vi "UHR-Fleezers Control (host) - 11.9b.vi"() -> ()   [LabVIEW 2014] (continued)
                                n672 = Multiply(x=w983, y=w984) -> (x*y=w982:dbl)
                                n673 = Round Toward -Infinity(1:w982) -> (0:w981:dbl)
                                n674 = Select(t=w981, s="Random Choice", f=w987) -> (s? t:f=w985:dbl)
                                n675 = Select(t="Yank to Trap D (MHz)", s="Yank to which?", f="Yank to SP") -> (s? t:f=w978:dbl[])
                                n676 = Index Array(array=w978, index=w985) -> (element=w988:dbl)
                                n677 = case shown="False" "Yank to which?" {
                                tunnel: w988 -> [w989 w1016]
                                frame False {
                                n678 = flat-sequence {
                                tunnel: w989 -> [w990]
                                frame #0 {
                                n679 = property on="Trap Pos FB SP" class="DigNum (strict)"("Val(Sgnl)"=w990) -> ()  [unwired: 2 in, 2 out]
                                }
                                frame #1 {
                                n680 = Wait (ms)(milliseconds to wait=u32 700) -> ()  [unwired: 1 out]
                                }
                                frame #2 {
                                n681 = local read "Action (%)"() -> (w995:dbl)
                                n682 = Absolute Value(x=w995) -> (abs(x)=w994:dbl)
                                n683 = Greater?(x=w994, y=70.0) -> (0:w992:bool)
                                n684 = property on="Remove Action Offset" class="Bool (strict)"("Val(Sgnl)"=w992) -> ()  [unwired: 2 in, 2 out]
                                }
                                frame #3 {
                                n685 = for {
                                N: 4 -> [_]
                                n686 = flat-sequence {
                                frame #0 {
                                n687 = Wait (ms)(milliseconds to wait=u32 500) -> ()  [unwired: 1 out]
                                }
                                frame #1 {
                                n688 = local read "Action (%)"() -> (w1001:dbl)
                                n689 = Absolute Value(x=w1001) -> (abs(x)=w1000:dbl)
                                n690 = Greater?(x=w1000, y=70.0) -> (0:w998:bool)
                                n691 = property on="Remove Action Offset" class="Bool (strict)"("Val(Sgnl)"=w998) -> ()  [unwired: 2 in, 2 out]
                                }
                                }
                                }
                                }
                                frame #4 {
                                n692 = local read "Shift confocal"() -> (w1005:bool)
                                n693 = local read "Mean"() -> (w1008:dbl)
                                n694 = Greater?(x=w1008, y=11.0) -> (0:w1004:bool)
                                n695 = Not(x=w1004) -> (.not. x?=w1003:bool)
                                n696 = And(x=w1003, y=w1005) -> (x .and. y?=w1002:bool)
                                n697 = And(x=w1004, y=w1005) -> (x .and. y?=w1006:bool)
                                n698 = case shown="True" w1006 {
                                frame False {
                                }
                                frame True {
                                n699 = local read "Confocal X 2 (V)"() -> (w1011:dbl)
                                n700 = local read "Confocal Y 2 (V)"() -> (w1012:dbl)
                                n701 = property on="AO2" class="Slide (strict)"("Val(Sgnl)"=w1011) -> ()  [unwired: 2 in, 2 out]
                                n702 = property on="AO1" class="Slide (strict)"("Val(Sgnl)"=w1012) -> ()  [unwired: 2 in, 2 out]
                                }
                                }
                                n703 = case shown="True" w1002 {
                                frame False {
                                }
                                frame True {
                                n704 = local read "Confocal X 1 (V)"() -> (w1009:dbl)
                                n705 = local read "Confocal Y 1 (V)"() -> (w1010:dbl)
                                n706 = property on="AO1" class="Slide (strict)"("Val(Sgnl)"=w1010) -> ()  [unwired: 2 in, 2 out]
                                n707 = property on="AO2" class="Slide (strict)"("Val(Sgnl)"=w1009) -> ()  [unwired: 2 in, 2 out]
                                }
                                }
                                }
                                frame #5 {
                                n708 = Wait (ms)(milliseconds to wait=u32 1500) -> ()  [unwired: 1 out]
                                }
                                frame #6 {
                                n709 = property on="Remove Offset" class="Bool (strict)"("Val(Sgnl)"=TRUE ("Value (Signaling)")) -> ()  [unwired: 2 in, 2 out]
                                n710 = property on="Rem fb disp offset" class="Bool (strict)"("Val(Sgnl)"=TRUE ("Value (Signaling)")) -> ()  [unwired: 2 in, 2 out]
                                }
                                }
                                }
                                frame True {
                                n711 = flat-sequence {
                                tunnel: w1016 -> [w1017]
                                frame #0 {
                                n712 = property on="Trap D (MHz)" class="DigNum (strict)"("Val(Sgnl)"=w1017) -> ()  [unwired: 2 in, 2 out]
                                }
                                frame #1 {
                                n713 = Wait (ms)(milliseconds to wait=u32 500) -> ()  [unwired: 1 out]
                                }
                                frame #2 {
                                n714 = local read "Shift confocal"() -> (w1021:bool)
                                n715 = local read "Mean"() -> (w1019:dbl)
                                n716 = Greater?(x=w1019, y=11.0) -> (0:w1022:bool)
                                n717 = Not(x=w1022) -> (.not. x?=w1023:bool)
                                n718 = And(x=w1023, y=w1021) -> (x .and. y?=w1025:bool)
                                n719 = And(x=w1022, y=w1021) -> (x .and. y?=w1024:bool)
                                n720 = case shown="True" w1024 {
                                frame False {
                                }
                                frame True {
                                n721 = local read "Confocal Y 2 (V)"() -> (w1029:dbl)
                                n722 = local read "Confocal X 2 (V)"() -> (w1028:dbl)
                                n723 = property on="AO1" class="Slide (strict)"("Val(Sgnl)"=w1029) -> ()  [unwired: 2 in, 2 out]
                                n724 = property on="AO2" class="Slide (strict)"("Val(Sgnl)"=w1028) -> ()  [unwired: 2 in, 2 out]
                                }
                                }
                                n725 = case shown="True" w1025 {
                                frame False {
                                }
                                frame True {
                                n726 = local read "Confocal X 1 (V)"() -> (w1026:dbl)
                                n727 = local read "Confocal Y 1 (V)"() -> (w1027:dbl)
                                n728 = property on="AO2" class="Slide (strict)"("Val(Sgnl)"=w1026) -> ()  [unwired: 2 in, 2 out]
                                n729 = property on="AO1" class="Slide (strict)"("Val(Sgnl)"=w1027) -> ()  [unwired: 2 in, 2 out]
                                }
                                }
                                }
                                }
                                }
                                }
                                }
                              }
                            }
                            frame "Raster" {
                              n730 = property on="Trap Raster Scan" class="Bool (strict)"("Val(Sgnl)"=TRUE ("Value (Signaling)")) -> ()  [unwired: 2 in, 2 out]
                            }
                          }
                          n731 = local read "Time (s)"() -> (w962:dbl)
                          "Fl. High" <- TRUE ("Yanking")
                        }
                        frame #1 {
                          n732 = local read "Auto F Reset"() -> (w1031:bool)
                          n733 = case shown="True" w1031 {
                            tunnel: w1036 -> [_ w1040]
                            tunnel: w1035 -> [_ w1039]
                            tunnel: w1034 -> [_ w1038]
                            tunnel: w1032 -> [_ w1037]
                            frame False {
                            }
                            frame True {
                              n734 = node-c288() -> (w1042:T21)  [unwired: 4 out]
                              n735 = timed-loop {
                                timing: w1042 -> [_]
                                timing-out: [_] -> w1041
                                tunnel: w1040 -> [w1060]
                                tunnel: w1039 -> [w1059]
                                tunnel: w1038 -> [w1058]
                                tunnel: w1037 -> [w1057]
                                stop <- w1043 stop-if-true
                                n736 = node-c288() -> ()  [unwired: 2 out]
                                n737 = local read "Fl. D Thresh. (kHz)"() -> (w1051:dbl)
                                n738 = local read "Fl. Triggered..."() -> (w1056:bool)
                                n739 = local read "Delta Fl. 1"() -> (w1047:dbl)
                                n740 = local read "Delta Fl. 2"() -> (w1045:dbl)
                                n741 = local read "Stop All"() -> (w1054:bool)
                                n742 = local read "APD to Watch"() -> (w1046:bool)
                                n743 = Select(t=w1047, s=w1046, f=w1045) -> (s? t:f=w1044:dbl)
                                n744 = Not(x=w1056) -> (.not. x?=w1055:bool)
                                n745 = Multiply(x=w1051, y=1000.0) -> (x*y=w1050:dbl)
                                n746 = Negate(x=w1050) -> (-x=w1049:dbl)
                                n747 = Less?(x=w1044, y=w1049) -> (x < y?=w1053:bool)
                                n748 = Compound Arithmetic op=OR(w1053, w1054, w1055, "Reset Force") -> (w1043:bool)
                                n749 = case shown="True" w1043 {
                                tunnel: w1060 -> [_ w1075]
                                tunnel: w1059 -> [_ w1074]
                                tunnel: w1058 -> [_ w1064]
                                tunnel: w1057 -> [_ w1066]
                                frame False {
                                }
                                frame True {
                                n750 = local read "Time (s)"() -> (w1065:dbl)
                                n751 = case shown="\"Yank\"" w1074 {
                                tunnel: w1075 -> [_ w1078]
                                tunnel: w1066 -> [_ w1076]
                                frame "Image", Default {
                                }
                                frame "Yank" {
                                n752 = flat-sequence {
                                tunnel: [w1084] -> w1079
                                tunnel: w1078 -> [w1084]
                                tunnel: [w1080] -> w1077
                                tunnel: w1076 -> [w1080]
                                tunnel: w1079 -> [w1087]
                                tunnel: w1077 -> [w1085]
                                frame #0 {
                                n753 = local read "Yank Delay (s)"() -> (w1083:dbl)
                                n754 = Multiply(x=w1083, y=1000.0) -> (x*y=w1081:dbl)
                                n755 = Wait (ms)(milliseconds to wait=w1081) -> ()  [unwired: 1 out]
                                }
                                frame #1 {
                                n756 = local read "Yank to which?"() -> (w1086:bool)
                                n757 = case shown="False" w1086 {
                                tunnel: w1087 -> [_ w1115]
                                tunnel: w1085 -> [w1088 _]
                                frame False {
                                n758 = flat-sequence {
                                tunnel: w1088 -> [w1089]
                                frame #0 {
                                n759 = property on="Trap Pos FB SP" class="DigNum (strict)"("Val(Sgnl)"=w1089) -> ()  [unwired: 2 in, 2 out]
                                }
                                frame #1 {
                                n760 = Wait (ms)(milliseconds to wait=u32 700) -> ()  [unwired: 1 out]
                                }
                                frame #2 {
                                n761 = local read "Action (%)"() -> (w1094:dbl)
                                n762 = Absolute Value(x=w1094) -> (abs(x)=w1093:dbl)
                                n763 = Greater?(x=w1093, y=70.0) -> (0:w1091:bool)
                                n764 = property on="Remove Action Offset" class="Bool (strict)"("Val(Sgnl)"=w1091) -> ()  [unwired: 2 in, 2 out]
                                }
                                frame #3 {
                                n765 = for {
                                N: 4 -> [_]
                                n766 = flat-sequence {
                                frame #0 {
                                n767 = Wait (ms)(milliseconds to wait=u32 500) -> ()  [unwired: 1 out]
                                }
                                frame #1 {
                                n768 = local read "Action (%)"() -> (w1100:dbl)
                                n769 = Absolute Value(x=w1100) -> (abs(x)=w1099:dbl)
                                n770 = Greater?(x=w1099, y=70.0) -> (0:w1097:bool)
                                n771 = property on="Remove Action Offset" class="Bool (strict)"("Val(Sgnl)"=w1097) -> ()  [unwired: 2 in, 2 out]
                                }
                                }
                                }
                                }
                                frame #4 {
                                n772 = local read "Shift confocal"() -> (w1105:bool)
                                n773 = local read "Mean"() -> (w1107:dbl)
                                n774 = Greater?(x=w1107, y=11.0) -> (0:w1104:bool)
                                n775 = Not(x=w1104) -> (.not. x?=w1103:bool)
                                n776 = And(x=w1104, y=w1105) -> (x .and. y?=w1102:bool)
                                n777 = And(x=w1103, y=w1105) -> (x .and. y?=w1101:bool)
                                n778 = case shown="True" w1102 {
                                frame False {
                                }
                                frame True {
                                n779 = local read "Confocal Y 2 (V)"() -> (w1111:dbl)
                                n780 = local read "Confocal X 2 (V)"() -> (w1110:dbl)
                                n781 = property on="AO2" class="Slide (strict)"("Val(Sgnl)"=w1110) -> ()  [unwired: 2 in, 2 out]
                                n782 = property on="AO1" class="Slide (strict)"("Val(Sgnl)"=w1111) -> ()  [unwired: 2 in, 2 out]
                                }
                                }
                                n783 = case shown="True" w1101 {
                                frame False {
                                }
                                frame True {
                                n784 = local read "Confocal X 1 (V)"() -> (w1108:dbl)
                                n785 = local read "Confocal Y 1 (V)"() -> (w1109:dbl)
                                n786 = property on="AO1" class="Slide (strict)"("Val(Sgnl)"=w1109) -> ()  [unwired: 2 in, 2 out]
                                n787 = property on="AO2" class="Slide (strict)"("Val(Sgnl)"=w1108) -> ()  [unwired: 2 in, 2 out]
                                }
                                }
                                }
                                frame #5 {
                                n788 = Wait (ms)(milliseconds to wait=u32 1500) -> ()  [unwired: 1 out]
                                }
                                frame #6 {
                                n789 = property on="Rem fb disp offset" class="Bool (strict)"("Val(Sgnl)"=TRUE ("Value (Signaling)")) -> ()  [unwired: 2 in, 2 out]
                                n790 = property on="Remove Offset" class="Bool (strict)"("Val(Sgnl)"=TRUE ("Value (Signaling)")) -> ()  [unwired: 2 in, 2 out]
                                }
                                }
                                }
                                frame True {
                                n791 = flat-sequence {
                                tunnel: w1115 -> [w1116]
                                frame #0 {
                                n792 = property on="Trap D (MHz)" class="DigNum (strict)"("Val(Sgnl)"=w1116) -> ()  [unwired: 2 in, 2 out]
                                }
                                frame #1 {
                                n793 = Wait (ms)(milliseconds to wait=u32 500) -> ()  [unwired: 1 out]
                                }
                                frame #2 {
                                n794 = local read "Shift confocal"() -> (w1122:bool)
                                n795 = local read "Mean"() -> (w1124:dbl)
                                n796 = Greater?(x=w1124, y=11.0) -> (0:w1121:bool)
                                n797 = Not(x=w1121) -> (.not. x?=w1120:bool)
                                n798 = And(x=w1121, y=w1122) -> (x .and. y?=w1119:bool)
                                n799 = And(x=w1120, y=w1122) -> (x .and. y?=w1118:bool)
                                n800 = case shown="True" w1119 {
                                frame False {
                                }
                                frame True {
                                n801 = local read "Confocal Y 2 (V)"() -> (w1128:dbl)
                                n802 = local read "Confocal X 2 (V)"() -> (w1127:dbl)
                                n803 = property on="AO2" class="Slide (strict)"("Val(Sgnl)"=w1127) -> ()  [unwired: 2 in, 2 out]
                                n804 = property on="AO1" class="Slide (strict)"("Val(Sgnl)"=w1128) -> ()  [unwired: 2 in, 2 out]
                                }
                                }
                                n805 = case shown="True" w1118 {
                                frame False {
                                }
                                frame True {
                                n806 = local read "Confocal Y 1 (V)"() -> (w1126:dbl)
                                n807 = local read "Confocal X 1 (V)"() -> (w1125:dbl)
                                n808 = property on="AO2" class="Slide (strict)"("Val(Sgnl)"=w1125) -> ()  [unwired: 2 in, 2 out]
                                n809 = property on="AO1" class="Slide (strict)"("Val(Sgnl)"=w1126) -> ()  [unwired: 2 in, 2 out]
                                }
                                }
                                }
                                }
                                }
                                }
                                }
                                }
                                }
                                }
                                n810 = local read "Messages"() -> (w1073:string)
                                n811 = Subtract(x=w1065, y=w1064) -> (x-y=w1071:dbl)
                                "Duration (s)" <- w1071
                                n812 = Number To Decimal String(number=w1071, width (-)=i16 0) -> (decimal integer string=w1069:string)
                                n813 = Concatenate Strings(w1069, " s fluorescence event." ("string")) -> (w1067:string)
                                n814 = call "Update messages.vi"("Message to add"=w1067, "Old message string"=w1073) -> ("New message string"=w1072:string)
                                n815 = local write "Reset Force"(FALSE ("Reset Force")) -> ()
                                n816 = local write "Waiting"(TRUE ("Waiting")) -> ()
                                n817 = local write "Messages"(w1072) -> ()
                                n818 = local write "Fl. High"(FALSE ("Fl. High")) -> ()
                                n819 = call <vilib>:"Beep.vi"() -> ()  [unwired: 3 in, 9 out]
                                }
                                }
                                n820 = node-c288() -> ()  [unwired: 2 out]
                              }
                              n821 = node-c288(w1041) -> ()  [unwired: 1 out]
                            }
                          }
                        }
                      }
                      n822 = local read "Trap Pos FB SP"() -> (w949:fxp<+/-,16,1>)
                      n823 = local read "Trap D (MHz)"() -> (w954:dbl)
                    }
                  }
                }
                frame #1 {
                  n824 = local read "Stop All"() -> (w1138:bool)
                  n825 = local read "Fl. Triggered..."() -> (w1136:bool)
                  n826 = Not(x=w1136) -> (.not. x?=w1137:bool)
                  n827 = Or(x=w1137, y=w1138) -> (x .or. y?=w1135:bool)
                }
              }
              n828 = case shown="True" w724 {
                frame False {
                }
                frame True {
                  n829 = local read "Confocal Y 1 (V)"() -> (w734:dbl)
                  n830 = local read "Confocal X 1 (V)"() -> (w733:dbl)
                  n831 = property on="AO2" class="Slide (strict)"("Val(Sgnl)"=w733) -> ()  [unwired: 2 in, 2 out]
                  n832 = property on="AO1" class="Slide (strict)"("Val(Sgnl)"=w734) -> ()  [unwired: 2 in, 2 out]
                }
              }
              n833 = case shown="True" w724 {
                frame False {
                }
                frame True {
                  w732 = FALSE ("Fl. High")
                  n834 = local write "Waiting"(w732) -> ()
                  n835 = local write "Fl. High"(w732) -> ()
                }
              }
              n836 = node-c288() -> ()  [unwired: 2 out]
            }
            n837 = node-c288(w722) -> ()  [unwired: 1 out]
          }
        }
      }
      event "Stop All": Value Change {
        n838 = event-data() -> ()  [unwired: 7 out]
        n839 = local read "Stop All"() -> (w1143:bool)
      }
    }
    n840 = node-c288() -> ()  [unwired: 2 out]
  }
  n841 = property on="Saved trap pos" class="WFGraph (strict)"("Visible"=TRUE) -> ()  [unwired: 2 in, 2 out]
  n842 = property on="Trap Delta Graph" class="WFGraph (strict)"("Visible"=FALSE) -> ()  [unwired: 2 in, 2 out]
  n843 = local write "Trap pos"(TRUE ("Trap pos")) -> ()
  n844 = node-c288(2 ("Processor")) -> (w113:T21)  [unwired: 3 out]
  n845 = timed-loop "Control parameters (event loop)" {
    tunnel: w23 -> [w1152]
    shift-right: [w1151] -> _
    shift-left: errorcluster {"status"=FALSE, "code"=0, "source"=""} ("error out") -> [w1150]
    tunnel: [w1149] -> _
    timing: w113 -> [_]
    timing-out: [_] -> w112
    tunnel: w86 -> [w1148]
    tunnel: w27 -> [w1147]
    tunnel: w26 -> [w1146]
    tunnel: w25 -> [w1145]
    tunnel: w24 -> [w1144]
    stop <- w1149 stop-if-true
    n846 = node-c288() -> ()  [unwired: 2 out]
    n847 = event shown="[20] \"Green laser mode\", \"Green ON/Interlacing\": Value Change" {
      selector: _ -> [_ _ _ _ _ _ _ _ _ _ _ _ _ _ _ _ _ _ _ _ _ _ _ _ _ _ _ _ _ _ _ _ _ _ _ _ _ _ _ _ _ _ _ _ _ _ _ _ _ _ _ _ _ _ _ _ _ _ _ _ _ _ _ _ _ _ _ _ _ _ _ _ _ _ _ _ _ _ _ _]
      dyn-events: _ -> [_ _ _ _ _ _ _ _ _ _ _ _ _ _ _ _ _ _ _ _ _ _ _ _ _ _ _ _ _ _ _ _ _ _ _ _ _ _ _ _ _ _ _ _ _ _ _ _ _ _ _ _ _ _ _ _ _ _ _ _ _ _ _ _ _ _ _ _ _ _ _ _ _ _ _ _ _ _ _ _]
      timeout: _ -> [_ _ _ _ _ _ _ _ _ _ _ _ _ _ _ _ _ _ _ _ _ _ _ _ _ _ _ _ _ _ _ _ _ _ _ _ _ _ _ _ _ _ _ _ _ _ _ _ _ _ _ _ _ _ _ _ _ _ _ _ _ _ _ _ _ _ _ _ _ _ _ _ _ _ _ _ _ _ _ _]
      tunnel: w1152 -> [w1190 _ _ _ w1228 _ w1250 _ _ _ _ w1316 _ _ w1359 w1365 w1370 w1376 w1412 w1430 w1439 _ w1456 w1460 w1471 w1482 w1493 w1504 w1515 w1526 w1553 w1647 w1654 w1692 _ _ w1752 w1756 w1767 w1771 w1775 _ w1783 _ _ _ _ _ _ _ _ _ _ _ _ _ _ _ _ _ w2164 _ w2181 _ w2188 w2206 _ w2213 w2221 w2236 w2247 w2253 _ w2262 _ w2281 _ _ _ w2356]
      tunnel: [w1189 _ _ _ w1218 _ w1249 _ _ w1281 _ w1295 _ _ w1358 w1361 w1367 w1373 w1411 w1428 w1438 _ w1454 _ w1465 w1476 w1487 w1498 w1509 w1520 w1551 w1645 w1652 w1690 _ _ w1750 w1754 w1757 w1769 w1773 _ w1781 _ _ _ _ _ _ _ _ _ _ _ _ _ _ _ _ _ w2162 _ _ _ _ w2203 _ _ _ _ _ _ _ _ _ _ _ _ _ w2354] -> w1151
      tunnel: w1150 -> [w1188 _ _ _ w1227 _ w1248 _ _ w1281 _ w1315 _ _ w1357 w1360 w1366 w1372 w1410 w1429 w1437 _ w1455 w1459 w1470 w1481 w1492 w1503 w1514 w1525 w1552 w1646 w1653 w1691 _ _ w1751 w1755 w1766 w1770 w1774 _ w1782 _ _ _ _ _ _ _ _ _ _ _ _ _ _ _ _ _ w2163 _ w2180 _ w2187 w2205 _ w2212 w2220 w2235 w2246 w2252 _ w2261 _ w2280 _ _ _ w2355]
      tunnel: [_ _ _ _ _ _ _ _ _ w1280 _ _ _ _ _ _ _ _ _ _ _ _ _ _ _ _ _ _ _ _ _ _ _ _ _ _ _ _ _ _ _ _ _ _ _ _ _ _ _ _ _ _ _ _ _ _ _ _ _ _ _ _ _ _ _ _ _ _ _ _ _ _ _ _ _ _ _ _ _ _] -> w1149
      tunnel: [_ _ _ _ _ _ _ "Round T1 X" _ _ _ _ _ _ _ _ _ _ _ _ _ _ _ _ _ _ _ _ _ _ _ _ _ _ _ _ _ _ _ _ _ _ _ _ _ _ _ _ _ _ _ _ _ _ _ _ _ _ _ _ _ _ _ _ _ _ _ _ _ _ _ _ _ _ _ _ _ _ _ _] -> _
      tunnel: [_ _ _ "Adjust Scale\nto Mean" _ _ _ _ _ _ _ _ _ _ _ _ _ _ _ _ _ _ "Test ttrig" _ _ _ _ _ _ _ _ _ _ _ _ _ _ _ _ _ _ _ _ _ _ _ _ _ _ _ "Flush Sample" "Flush Pump 3" "Flush Pump 1" "Clear Volume" _ _ _ _ _ _ _ _ _ _ _ _ _ _ _ _ _ _ _ _ _ _ _ _ _ _] -> _
      tunnel: [_ _ _ _ _ _ _ _ "Round T2 X" _ "Delayed Interlace Start" _ _ _ _ _ _ _ _ _ _ _ _ _ _ _ _ _ _ _ _ _ _ _ _ _ _ _ _ _ _ _ _ _ _ _ _ _ _ _ _ _ _ _ _ _ _ _ _ _ _ _ _ _ _ _ _ _ _ _ _ _ _ _ _ _ _ _ _ _] -> _
      tunnel: w1148 -> [_ _ _ _ _ _ _ _ _ _ _ _ _ _ _ _ _ _ _ _ _ _ _ _ _ _ _ _ _ _ _ _ _ _ _ _ _ _ _ _ _ _ _ _ _ _ w1941 w1959 w1966 w1971 w1977 _ _ w2076 _ _ _ _ _ _ _ _ _ _ _ _ _ _ _ _ _ _ _ _ _ _ _ _ _ _]
      tunnel: w1147 -> [_ _ _ _ _ _ _ _ _ _ _ _ _ _ _ _ _ _ _ _ _ _ _ _ _ _ _ _ _ _ _ _ _ _ _ _ _ _ _ _ _ _ _ _ w1857 _ _ _ _ _ _ w2007 _ _ w2083 _ w2092 _ w2106 _ _ _ _ _ _ _ _ _ _ _ _ _ _ _ _ _ _ _ _ _]
      tunnel: w1146 -> [_ _ _ _ _ _ _ _ _ _ _ _ _ _ _ _ _ _ _ _ _ _ _ _ _ _ _ _ _ _ _ _ _ _ _ _ _ _ _ _ _ _ _ _ _ _ _ _ _ _ _ _ _ _ _ _ _ _ _ _ _ _ _ _ _ _ _ _ _ _ _ _ _ _ _ _ _ _ _ _]
      tunnel: w1145 -> [_ _ _ _ _ _ _ _ _ _ _ _ _ _ _ _ _ _ _ _ _ _ _ _ _ _ _ _ _ _ _ _ _ _ _ _ _ _ _ _ _ _ _ w1794 _ _ _ _ _ _ _ _ w2037 _ _ w2088 _ w2099 _ w2131 _ _ _ _ _ _ _ _ _ _ _ _ _ _ _ _ _ _ _ _]
      tunnel: w1144 -> [_ _ _ _ _ _ _ _ _ _ _ _ _ _ _ _ _ _ _ _ _ _ _ _ _ _ _ _ _ _ _ _ _ _ _ _ _ _ _ _ _ _ _ _ _ _ _ _ _ _ _ _ _ _ _ _ _ _ _ _ _ _ _ _ _ _ _ _ _ _ _ _ _ _ _ _ _ _ _ _]
      event "AI Count (ticks)", "Sets to FIFO (Traps)", "Save ave N", "FPGA Ave.", "# Samples/channel", "N sets to save": Value Change {
        # "So that if 'Save ave N' is updated, the AOD scanning code updates too."
        n848 = event-data() -> ()  [unwired: 6 out]
        n849 = local read "AI Count (ticks)"() -> (w1170:u32)
        n850 = Boolean To (0,1)(Boolean="Sets to FIFO (Traps)") -> (0, 1=w1180:cluster{"Set 1":i16, "Set 2":i16, "Set 3":i16})
        n851 = Cluster To Array(cluster=w1180) -> (array=w1179:i16[])
        n852 = xnode "Read/Write Control"("FPGA VI Reference In"=w1190, "error in"=w1188, "ai count"=w1170, "AI1 Sets to FIFO"="Sets to FIFO (Traps)", "N of AI1 Int Acq Sets"="N Acq Sets (Traps + Fl.)") -> ("error out"=w1189:errorcluster)  [unwired: 1 out]
        n853 = To Unsigned Long Integer(number=w1179) -> (unsigned 32bit integer=w1159:u32[])
        n854 = local read "Scan steps (AOD)"() -> (w1181:u64)
        n855 = Multiply(x=w1170, y="N Acq Sets (Traps + Fl.)") -> (x*y=w1168:u32)
        n856 = Divide(x=40000000.0, y=w1170) -> (x/y=w1162:dbl)
        "AI rate (Hz)" <- w1162
        "Ave. Rate (Hz)" <- w1162
        n857 = Add Array Elements(numeric array=w1159) -> (sum=w1171:u32)
        "Trap Sets" <- w1171
        n858 = Reciprocal(x=w1162) -> (1/x=→"Ave. Period (s)":dbl)
        n859 = property on="Scan steps (AOD)" class="DigNum (strict)"("Val(Sgnl)"=w1181) -> ()  [unwired: 2 in, 2 out]
        n860 = Divide(x=w1162, y="N Acq Sets (Traps + Fl.)") -> (x/y=w1185:dbl)
        "Data Rate (Hz)" <- w1185
        n861 = Reciprocal(x=w1185) -> (1/x=→"Data Period (s)":dbl)
        n862 = local read "Save ave N"() -> (w1184:dbl)
        n863 = Divide(x=w1185, y=w1184) -> (x/y=w1183:dbl)
        "Save Data Rate (Hz)" <- w1183
        n864 = Reciprocal(x=w1183) -> (1/x=→"Save Data Period (s)":dbl)
        n865 = Multiply(x=w1168, y="# Samples/trap") -> (x*y=w1166:u32)
        "Counts/DMA" <- w1166
        n866 = property on="Trap Disp. Downsample" class="DigNum (strict)"("Maximum"="# Samples/trap") -> ()  [unwired: 2 in, 2 out]
        n867 = Multiply(x=w1171, y="# Samples/trap") -> (x*y=w1160:u32)
        "# Samples/channel" <- w1160
        n868 = Multiply(x=w1160, y=u32 8) -> (x*y=→"Trap AI Elements/DMA read":u32)
        n869 = local read "APD Int. Count"() -> (w1167:u32)
        n870 = Multiply(x=w1160, y=u32 3) -> (x*y=→"Trap Pos Elements/DMA read":u32)
        n871 = Divide(x=w1166, y=w1167) -> (x/y=w1157:dbl)
        "APD Samples/FIFO Acq." <- w1157
        n872 = Divide(x=w1166, y=40000000.0) -> (x/y=w1164:dbl)
        "DMA Update Period (s)" <- w1164
        n873 = Multiply(x=2.0, y=w1157) -> (x*y=→"APD Elements/DMA read":dbl)
        n874 = property on="APD Disp. Downsample" class="DigNum (strict)"("Maximum"=w1157) -> ()  [unwired: 2 in, 2 out]
        n875 = local read "N sets to save"() -> (w1177:u32)
        n876 = Multiply(x=w1164, y=w1177) -> (x*y=→"Total Time (s)":dbl)
        "FPGA Averaging" <- FALSE ("FPGA Averaging")
      }
      event "Remove Offset": Value Change {
        n877 = event-data() -> ()  [unwired: 7 out]
        n878 = local write "Remove Offset"(FALSE ("Remove Offset")) -> ()
        n879 = local read "Bead Mean (nm)"() -> (w1192:dbl)
        n880 = local read "Offset (nm)"() -> (w1193:dbl)
        n881 = Add(x=w1192, y=w1193) -> (x+y=w1191:dbl)
        n882 = local write "Offset (nm)"(w1191) -> ()
        n883 = disable-structure shown="Disabled" {
          frame Disabled {
            n884 = local read "Bead Mean (nm)"() -> (w1198:dbl)
            n885 = Add(y=w1198) -> (x=w1197:dbl, x+y=w1196:dbl)
            n886 = Subtract(x=w1198, y=w1197) -> (x-y=w1195:dbl)
            n887 = property on="Bead Separation" class="WFChart (strict)"("YScale.Minimum"=w1195) -> ()  [unwired: 2 in, 2 out]
            n888 = property on="Bead Separation" class="WFChart (strict)"("YScale.Maximum"=w1196) -> ()  [unwired: 2 in, 2 out]
          }
          frame Enabled {
          }
        }
      }
      event "Detector Type": Value Change {
        n889 = event-data() -> ()  [unwired: 7 out]
        n890 = local read "AI labels"() -> (w1199:string[])
        n891 = property on="High Res. Display" class="Ring (strict)"("Strings []"=w1199) -> ()  [unwired: 2 in, 2 out]
        n892 = Build Array (concatenate)(w1199, "none") -> (w1200:string[])
        n893 = property on="FFT 1 Choice 1" class="Ring (strict)"("Strings []"=w1200) -> ()  [unwired: 2 in, 2 out]
        n894 = property on="FFT 1 Choice 2" class="Ring (strict)"("Strings []"=w1200) -> ()  [unwired: 2 in, 2 out]
        n895 = property on="FFT 2 Choice 1" class="Ring (strict)"("Strings []"=w1200) -> ()  [unwired: 2 in, 2 out]
        n896 = property on="FFT 2 Choice 2" class="Ring (strict)"("Strings []"=w1200) -> ()  [unwired: 2 in, 2 out]
        n897 = Bundle("APD 1", "APD 2") -> (w1203:cluster{string, string})  [unwired: 1 out]
        n898 = Cluster To Array(cluster=w1203) -> (array=w1201:string[])
        n899 = Build Array (concatenate)(w1201, w1200) -> (w1205:string[])
        n900 = Array Size(array=w1205) -> (size(s)=w1206:i32)
        n901 = property on="Signals to Plot" class="LstBox (strict)"("Item Names"=w1205) -> ()  [unwired: 2 in, 2 out]
        n902 = property on="Signals to Plot" class="LstBox (strict)"("Number of Rows"=w1206) -> ()  [unwired: 2 in, 2 out]
        n903 = property on="All Signals" class="WFChart (strict)"("LegNumRows"=w1206) -> ()  [unwired: 2 in, 2 out]
      }
      event "Adjust Scale\nto Mean": Value Change {
        n904 = event-data() -> ()  [unwired: 7 out]
        n905 = local read "APD 1 Rate (Hz)"() -> (w1215:dbl)
        n906 = Multiply(x=1000.0, y="Above (kHz)") -> (x*y=w1213:dbl)
        n907 = Multiply(x=1000.0, y="Below (kHz)") -> (x*y=w1211:dbl)
        n908 = Add(x=w1213, y=w1215) -> (x+y=w1208:dbl)
        n909 = Subtract(x=w1215, y=w1211) -> (x-y=w1209:dbl)
        n910 = property on="APD Chart" class="WFChart (strict)"("YScale.Minimum"=w1209) -> ()  [unwired: 2 in, 2 out]
        n911 = property on="APD Chart" class="WFChart (strict)"("YScale.Maximum"=w1208) -> ()  [unwired: 2 in, 2 out]
      }
      event "Phase adj. (AI1)", "+ phase (AI1)", "- phase (AI1)": Value Change {
        n912 = event-data() -> ()  [unwired: 7 out]
        n913 = Negate(x="Phase adj. (AI1)") -> (-x=w1225:i16)
        n914 = Select(t=w1225, s="- phase (AI1)", f="Phase adj. (AI1)") -> (s? t:f=w1224:i16)
        n915 = xnode "Read/Write Control"("FPGA VI Reference In"=w1228, "error in"=w1227, "Phase count adjustment"=w1224) -> ("FPGA VI Reference Out"=w1223:T19, "error out"=w1222:errorcluster)
        n916 = Or(x="- phase (AI1)", y="+ phase (AI1)") -> (x .or. y?=w1219:bool)
        n917 = xnode "Read/Write Control"("FPGA VI Reference In"=w1223, "error in"=w1222, "+ phase"=w1219) -> ("error out"=w1218:errorcluster)  [unwired: 1 out]
      }
      event "Signals to Plot": Double Click {
        w1231 = u32 9868950 ("Color Box")
        n918 = event-data() -> ("Row"=w1233:i32)  [unwired: 9 out]
        n919 = property on="All Signals" class="WFChart (strict)"("Active Plot"=w1233) -> (error out=w1244:errorcluster)  [unwired: 2 in, 1 out]
        n920 = property on="All Signals" class="WFChart (strict)" props=["Plot", "Visible?", "Plot", "Plot Color"](error in=w1244) -> (error out=w1243:errorcluster, "Plot.Visible?"=w1242:bool)  [unwired: 1 in, 2 out]
        n921 = Select(t=FALSE ("Plot.Visible"), s=w1242, f=TRUE ("Plot.Visible")) -> (s? t:f=w1237:bool)
        n922 = property on="All Signals" class="WFChart (strict)"(error in=w1243, "Plot.Visible?"=w1237) -> (error out=w1239:errorcluster)  [unwired: 1 in, 1 out]
        n923 = property on="All Signals" class="WFChart (strict)"(error in=w1239) -> (error out=w1234:errorcluster, "Plot.Plot Color"=w1238:u32)  [unwired: 1 in, 1 out]
        n924 = property on="Signals to Plot" class="LstBox (strict)"(error in=w1234, "Active Row"=w1233) -> (error out=w1232:errorcluster)  [unwired: 1 in, 1 out]
        n925 = Select(t=w1238, s=w1237, f=u32 0) -> (s? t:f=w1235:u32)
        n926 = property on="Signals to Plot" class="LstBox (strict)"(error in=w1232, "CellFontColor"=w1235, "SelColor"=w1231, "CellBG"=w1231, "CellFontSize"=u32 20 ("Active Row:Cell Font:Size"), "CellFontBold"=TRUE ("Active Row:Cell Font:Bold")) -> ()  [unwired: 1 in, 2 out]
      }
      event "BD 1 Frequency 1 (MHz)", "BD 1 Frequency 2 (MHz)", "BD 1 Frequency 3 (MHz)", "BD 2 Frequency 1 (MHz)", "BD 2 Frequency 2 (MHz)", "BD 2 Frequency 3 (MHz)", "Trap D (MHz)": Value Change {
        n927 = event-data() -> ("CtlRef"=w1247:refnum<vi>)  [unwired: 6 out]
        n928 = control-ref of="Trap D (MHz)"() -> (w1246:refnum<vi>)
        n929 = Equal?(x=w1246, y=w1247) -> (x = y?=w1245:bool)
        n930 = case shown="False" "Oscillate Set 1" {
          tunnel: w1250 -> [w1270 _]
          tunnel: [w1269 w1273] -> w1249
          tunnel: w1248 -> [w1268 w1273]
          tunnel: w1245 -> [w1253 _]
          frame False {
            n931 = local read "BD 1 Frequency 2 (MHz)"() -> (w1257:dbl)
            n932 = local read "BD 1 Frequency 1 (MHz)"() -> (w1255:dbl)
            n933 = Subtract(x=w1257, y="Trap D (MHz)") -> (x-y=w1254:dbl)
            n934 = Select(t=w1254, s=w1253, f=w1255) -> (s? t:f=w1252:dbl)
            n935 = local read "Y RF Frequency Limits (MHz)"() -> (w1258:T16)
            n936 = local read "X RF Frequency Limits (MHz)"() -> (w1259:T16)
            n937 = local read "BD 1 Frequency 3 (MHz)"() -> (w1271:dbl)
            n938 = local write "BD 1 Frequency 1 (MHz)"(w1252) -> ()
            n939 = local read "BD 2 Frequency 1 (MHz)"() -> (w1262:dbl)
            n940 = local read "BD 2 Frequency 2 (MHz)"() -> (w1261:dbl)
            n941 = local read "BD 2 Frequency 3 (MHz)"() -> (w1272:dbl)
            n942 = call "set RF board frequency - interlace.vi"("Board 2 Frequency Limits"=w1258, "Board 1 Frequency Limits"=w1259, "error in"=w1268, "FPGA VI Reference In"=w1270, "Board 2 Frequency 3 (MHz)"=w1272, "Board 1 Frequency 3 (MHz)"=w1271, "Board 2 Frequency 2 (MHz)"=w1261, "Board 2 Frequency 1 (MHz)"=w1262, "Board 1 Frequency 2 (MHz)"=w1257, "Board 1 Frequency 1  (MHz)"=w1252) -> ("error out"=w1269:errorcluster)  [unwired: 1 out]
            n943 = Subtract(x=w1262, y=w1261) -> (x-y=w1266:dbl)
            n944 = Subtract(x=w1252, y=w1257) -> (x-y=w1267:dbl)
            n945 = Square(x=w1266) -> (x^2=w1264:dbl)
            n946 = Square(x=w1267) -> (x^2=w1265:dbl)
            n947 = Add(x=w1265, y=w1264) -> (x+y=w1263:dbl)
            n948 = Square Root(x=w1263) -> (sqrt(x)=w1260:dbl)
            n949 = local write "Trap D (MHz)"(w1260) -> ()
            n950 = property on="Initial D (MHz)" class="DigNum (strict)"("Val(Sgnl)"=w1260) -> ()  [unwired: 2 in, 2 out]
          }
          frame True {
          }
        }
      }
      event "Round T1 X": Value Change {
        n951 = event-data() -> ()  [unwired: 7 out]
        n952 = local read "BD 1 Frequency 1 (MHz)"() -> (w1276:dbl)
        n953 = Round To Nearest(number=w1276) -> (nearest integer value=w1275:dbl)
        n954 = property on="BD 1 Frequency 1 (MHz)" class="DigNum (strict)"("Val(Sgnl)"=w1275) -> ()  [unwired: 2 in, 2 out]
      }
      event "Round T2 X": Value Change {
        n955 = event-data() -> ()  [unwired: 7 out]
        n956 = local read "BD 1 Frequency 2 (MHz)"() -> (w1278:dbl)
        n957 = Round To Nearest(number=w1278) -> (nearest integer value=w1277:dbl)
        n958 = property on="BD 1 Frequency 2 (MHz)" class="DigNum (strict)"("Val(Sgnl)"=w1277) -> ()  [unwired: 2 in, 2 out]
      }
      event "Stop All": Value Change {
        n959 = event-data() -> ()  [unwired: 7 out]
        n960 = local read "Stop All"() -> (w1280:bool)
      }
      event "Delayed Interlace Start": Value Change {
        n961 = event-data() -> ()  [unwired: 7 out]
        n962 = flat-sequence {
          frame #0 {
            n963 = Multiply(x="Delay to Interlace (s)", y=1000.0) -> (x*y=w1283:dbl)
            n964 = Wait (ms)(milliseconds to wait=w1283) -> ()  [unwired: 1 out]
          }
          frame #1 {
            n965 = property on="Green laser mode" class="RadioBtnsControl (strict)"("Val(Sgnl)"=enum32{"Laser ON", "Laser OFF", "Interlace"}."Interlace" ("Value (Signaling)")) -> ()  [unwired: 2 in, 2 out]
          }
        }
      }
      event "BD 1 Amplitude 1 (%)", "BD 1 Amplitude 2 (%)", "BD 1 Amplitude 3 (%)", "BD 2 Amplitude 1 (%)", "BD 2 Amplitude 2 (%)", "BD 2 Amplitude 3 (%)", "Trap 1 ON", "Trap 2 ON", "Trap 3 ON", "Feedback On/Off", "All FB On/Off": Value Change {
        w1307 = i16 1 ("f")
        n966 = event-data() -> ()  [unwired: 7 out]
        n967 = local write "Trap 1 (ON/OFF)"("Trap 1 ON") -> ()
        n968 = local write "Trap 2 (ON/OFF)"("Trap 2 ON") -> ()
        n969 = Boolean To (0,1)(Boolean="Trap 3 ON") -> (0, 1=w1308:i16)
        n970 = Boolean To (0,1)(Boolean="Trap 1 ON") -> (0, 1=w1309:i16)
        n971 = Boolean To (0,1)(Boolean="Trap 2 ON") -> (0, 1=w1310:i16)
        n972 = Select(t=w1310, s="Trap ON/OFF X or Y Amp?", f=w1307) -> (s? t:f=w1305:i16)
        n973 = Select(t=w1309, s="Trap ON/OFF X or Y Amp?", f=w1307) -> (s? t:f=w1306:i16)
        n974 = Select(t=w1308, s="Trap ON/OFF X or Y Amp?", f=w1307) -> (s? t:f=w1304:i16)
        n975 = Select(t=w1307, s="Trap ON/OFF X or Y Amp?", f=w1310) -> (s? t:f=w1302:i16)
        n976 = Select(t=w1307, s="Trap ON/OFF X or Y Amp?", f=w1309) -> (s? t:f=w1303:i16)
        n977 = Select(t=w1307, s="Trap ON/OFF X or Y Amp?", f=w1308) -> (s? t:f=w1301:i16)
        n978 = And(x="All FB On/Off", y="Feedback On/Off") -> (x .and. y?=w1299:cluster{"Set 1":bool, "Set 2":bool})
        n979 = local read "BD 1 Amplitude 1 (%)"() -> (w1319:dbl)
        n980 = local read "BD 1 Amplitude 2 (%)"() -> (w1318:dbl)
        n981 = local read "BD 1 Amplitude 3 (%)"() -> (w1317:dbl)
        n982 = Unbundle By Name(w1299) -> ("Set 1"=w1294:bool, "Set 2"=w1291:bool)
        n983 = local read "Y RF Amplitude Limits (%)"() -> (w1287:T16)
        n984 = local read "X RF Amplitude Limits (%)"() -> (w1288:T16)
        n985 = local read "BD 2 Amplitude 1 (%)"() -> (w1320:dbl)
        n986 = local read "BD 2 Amplitude 2 (%)"() -> (w1321:dbl)
        n987 = local read "BD 2 Amplitude 3 (%)"() -> (w1322:dbl)
        n988 = And(x="Trap 2 ON", y=w1291) -> (x .and. y?=w1289:bool)
        n989 = And(x="Trap 1 ON", y=w1294) -> (x .and. y?=w1292:bool)
        n990 = Multiply(x=w1306, y=w1319) -> (x*y=w1314:dbl)
        n991 = Multiply(x=w1318, y=w1305) -> (x*y=w1312:dbl)
        n992 = Multiply(x=w1317, y=w1304) -> (x*y=w1313:dbl)
        n993 = Multiply(x=w1320, y=w1303) -> (x*y=w1323:dbl)
        n994 = Multiply(x=w1321, y=w1302) -> (x*y=w1324:dbl)
        n995 = Multiply(x=w1322, y=w1301) -> (x*y=w1325:dbl)
        n996 = call "set RF board amplitude - interlace.vi"("Board 2 Amplitude Limits"=w1287, "Board 1 Amplitude Limits"=w1288, "error in"=w1315, "FPGA VI Reference In"=w1316, "Board 2 Amplitude 3 (%)"=w1325, "Board 1 Amplitude 3 (%)"=w1313, "Board 2 Amplitude 2 (%)"=w1324, "Board 2 Amplitude 1 (%)"=w1323, "Board 1 Amplitude 2 (%)"=w1312, "Board 1 Amplitude 1 (%)"=w1314) -> ("error out"=w1296:errorcluster, "FPGA VI Reference Out"=w1297:T19)
        n997 = xnode "Read/Write Control"("FPGA VI Reference In"=w1297, "error in"=w1296, "FB On/Off Set 1"=w1292, "FB On/Off Set 2"=w1289) -> ("error out"=w1295:errorcluster)  [unwired: 1 out]
      }
      event "Load parameters": Value Change {
        n998 = event-data() -> ()  [unwired: 7 out]
        n999 = property on="Saved AOD Raster Scan Parameter Sets" class="Arr (strict)"() -> ("Index Values"=w1336:u32[])  [unwired: 2 in, 2 out]
        n1000 = Index Array(array=w1336, index=0) -> (element=w1333:u32)
        n1001 = local write "Load parameters"(FALSE ("Load parameters")) -> ()
        n1002 = Index Array(array="Saved AOD Raster Scan Parameter Sets", index=w1333) -> (element=w1332:T26)
        n1003 = Unbundle By Name(w1332) -> ("Scan Range AOD (nm) 2"=w1331:dbl, "Step Size AOD (nm) 2"=w1330:dbl, "Scan Speed AOD (nm/s) 2"=w1329:dbl, "Number of scans (AOD) 2"=w1328:u16)
        n1004 = flat-sequence {
          tunnel: w1331 -> [w1339]
          tunnel: w1330 -> [w1338]
          tunnel: w1329 -> [w1337]
          tunnel: w1328 -> [w1340]
          frame #0 {
            n1005 = local write "Scan Speed (nm/s)"(w1337) -> ()
            n1006 = local write "Scan Range (nm)"(w1339) -> ()
            n1007 = local write "Step Size (nm)"(w1338) -> ()
          }
          frame #1 {
            n1008 = property on="Number of F/B Scans (AOD)" class="DigNum (strict)"("Val(Sgnl)"=w1340) -> ()  [unwired: 2 in, 2 out]
          }
        }
      }
      event "Trap 1 (ON/OFF)", "Trap 2 (ON/OFF)": Value Change {
        n1009 = event-data() -> ()  [unwired: 7 out]
        n1010 = property on="Trap 2 ON" class="Bool (strict)"("Val(Sgnl)"="Trap 2 (ON/OFF)") -> ()  [unwired: 2 in, 2 out]
        n1011 = property on="Trap 1 ON" class="Bool (strict)"("Val(Sgnl)"="Trap 1 (ON/OFF)") -> ()  [unwired: 2 in, 2 out]
      }
      event "DIO count 1 (ticks)", "DIO count 2 (ticks)", "DIO count 3 (ticks)", "Interlace", "Number Interlace Sets", "Not-Interlacing Set": Value Change {
        n1012 = event-data() -> ()  [unwired: 7 out]
        n1013 = local read "DIO count 3 (ticks)"() -> (w1353:u32)
        n1014 = local read "DIO count 1 (ticks)"() -> (w1355:u32)
        n1015 = local read "DIO count 2 (ticks)"() -> (w1354:u32)
        n1016 = To Unsigned Byte Integer(number="Not-Interlacing Set") -> (unsigned 8bit integer=w1344:u8)
        n1017 = Add(x=w1344, y=u8 1) -> (x+y=w1348:u8)
        n1018 = xnode "Read/Write Control"("FPGA VI Reference In"=w1359, "error in"=w1357, "DIO count 1 (ticks)"=w1355, "DIO count 2 (ticks)"=w1354, "DIO count 3 (ticks)"=w1353, "Interlace ON/OFF"="Interlace", "Number Interlace Cycles"="Number Interlace Sets", "Interlace Off Parameters"=w1348) -> ("error out"=w1358:errorcluster)  [unwired: 1 out]
        n1019 = Build Array(w1355, w1354, w1353) -> (w1346:u32[])
        n1020 = Split 1D Array(array=w1346, index="Number Interlace Sets") -> (first subarray=w1356:u32[])  [unwired: 1 out]
        n1021 = Index Array(array=w1346, index=w1344) -> (element=w1345:u32)
        n1022 = Add Array Elements(numeric array=w1356) -> (sum=w1350:u32)
        n1023 = Select(t=w1350, s="Interlace", f=w1345) -> (s? t:f=→"Total Counts (ticks)":u32)
      }
      event "Reset Feedback": Value Change {
        n1024 = event-data() -> ()  [unwired: 7 out]
        n1025 = Unbundle By Name("Reset Feedback") -> ("Set 1"=w1363:bool, "Set 2"=w1362:bool)
        n1026 = xnode "Read/Write Control"("FPGA VI Reference In"=w1365, "error in"=w1360, "FB Reset Set 1"=w1363, "FB Reset Set 2"=w1362) -> ("error out"=w1361:errorcluster)  [unwired: 1 out]
      }
      event "PID Gains": Value Change {
        n1027 = event-data() -> ()  [unwired: 7 out]
        n1028 = Unbundle By Name("PID Gains") -> ("Set 1"=w1369:T14, "Set 2"=w1368:T14)
        n1029 = xnode "Read/Write Control"("FPGA VI Reference In"=w1370, "error in"=w1366, "FB Gains Set 1"=w1369, "FB Gains Set 2"=w1368) -> ("error out"=w1367:errorcluster)  [unwired: 1 out]
      }
      event "AI2 to Setpoint", "Setpoints (V)": Value Change {
        n1030 = event-data() -> ()  [unwired: 7 out]
        n1031 = xnode "Read/Write Control"("FPGA VI Reference In"=w1376, "error in"=w1372) -> ("FPGA VI Reference Out"=w1375:T19, "error out"=w1374:errorcluster, "AI2 Y Sum Set 1"=w1383:i16, "AI2 Y Sum Set 2"=w1382:i16)
        n1032 = Cluster To Array(cluster="AI2 to Setpoint") -> (array=w1386:bool[])
        n1033 = local read "AI2 (V)"() -> (w1384:cluster{"Set 1":dbl, "Set 2":dbl})
        n1034 = Or Array Elements(Boolean array=w1386) -> (logical OR=w1387:bool)
        n1035 = Bundle By Name(cluster=w1384, "Set 1"=w1383, "Set 2"=w1382) -> (w1381:cluster{"Set 1":dbl, "Set 2":dbl})
        n1036 = Divide(x=w1381, y=3276.7) -> (x/y=w1380:cluster{"Set 1":dbl, "Set 2":dbl})
        "AI2 (V)" <- w1380
        n1037 = case shown="True" w1387 {
          tunnel: [w1390 w1407] -> w1379
          tunnel: "AI2 to Setpoint" -> [_ w1403]
          tunnel: "Setpoints (V)" -> [w1391 w1406]
          tunnel: w1380 -> [_ w1400]
          frame False {
            n1038 = Multiply(x=3276.7, y=w1391) -> (x*y=w1392:cluster{"Set 1":dbl, "Set 2":dbl})
            n1039 = To Word Integer(number=w1392) -> (16bit integer=w1390:cluster{"Set 1":i16, "Set 2":i16})
          }
          frame True {
            n1040 = Unbundle By Name(w1400) -> ("Set 1"=w1399:dbl, "Set 2"=w1398:dbl)
            n1041 = Unbundle By Name(w1406) -> ("Set 1"=w1405:dbl, "Set 2"=w1404:dbl)
            n1042 = Unbundle By Name(w1403) -> ("Set 1"=w1402:bool, "Set 2"=w1401:bool)
            n1043 = Select(t=w1399, s=w1402, f=w1405) -> (s? t:f=w1397:dbl)
            n1044 = Select(t=w1398, s=w1401, f=w1404) -> (s? t:f=w1396:dbl)
            n1045 = Bundle By Name(cluster=w1406, "Set 1"=w1397, "Set 2"=w1396) -> (w1394:cluster{"Set 1":dbl, "Set 2":dbl})
            n1046 = local write "Setpoints (V)"(w1394) -> ()
            n1047 = Multiply(x=3276.7, y=w1394) -> (x*y=w1395:cluster{"Set 1":dbl, "Set 2":dbl})
            n1048 = To Word Integer(number=w1395) -> (16bit integer=w1407:cluster{"Set 1":i16, "Set 2":i16})
          }
        }
        n1049 = Unbundle By Name(w1379) -> ("Set 1"=w1378:i16, "Set 2"=w1377:i16)
        n1050 = xnode "Read/Write Control"("FPGA VI Reference In"=w1375, "error in"=w1374, "FB Setpoint Set 1"=w1378, "FB Setpoint Set 2"=w1377) -> ("error out"=w1373:errorcluster)  [unwired: 1 out]
      }
      event "Invert GI": Value Change {
        n1051 = event-data() -> ()  [unwired: 7 out]
        n1052 = xnode "Read/Write Control"("FPGA VI Reference In"=w1412, "error in"=w1410, "Invert GI"="Invert GI", "Invert GI 2"="Invert GI") -> ("error out"=w1411:errorcluster)  [unwired: 1 out]
      }
      event "Green FB Setpoint (mV)", "Green FB Gains", "Green FB On/Off", "Current When FB OFF (%)", "Green int current ON count adj": Value Change {
        n1053 = event-data() -> ()  [unwired: 7 out]
        n1054 = local read "Green FB Setpoint (mV)"() -> (w1419:dbl)
        n1055 = local read "Current When FB OFF (%)"() -> (w1422:dbl)
        n1056 = Multiply(x=w1419, y=3.2767) -> (x*y=w1418:dbl)
        n1057 = Multiply(x=w1422, y=655.35) -> (x*y=w1423:dbl)
        n1058 = To Unsigned Word Integer(number=w1423) -> (unsigned 16bit integer=w1421:u16)
        n1059 = local read "Green int current ON count adj"() -> (w1426:u32)
        n1060 = local read "Green FB Gains"() -> (w1425:T14)
        n1061 = local read "Green ON/Interlacing"() -> (w1416:bool)
        n1062 = local read "Green laser mode"() -> (w1415:enum32{"Laser ON", "Laser OFF", "Interlace"})
        n1063 = local read "Green FB On/Off"() -> (w1427:bool)
        n1064 = Equal?(x=w1415, y=enum32{"Laser ON", "Laser OFF", "Interlace"}."Interlace") -> (x = y?=w1413:bool)
        n1065 = Compound Arithmetic op=AND(w1413, w1427, w1416) -> (w1417:bool)
        n1066 = xnode "Read/Write Control"("FPGA VI Reference In"=w1430, "error in"=w1429, "Green FB Setpoint"=w1418, "Green FB On/Off"=w1417, "Current Out"=w1421, "Green int current ON count adj"=w1426, "Green FB Gains"=w1425) -> ("error out"=w1428:errorcluster)  [unwired: 1 out]
      }
      event "Green laser mode", "Green ON/Interlacing": Value Change {
        n1067 = event-data() -> ()  [unwired: 7 out]
        n1068 = local write "Green Laser ON/OFF"("Green ON/Interlacing") -> ()
        n1069 = case shown="True" "Green ON/Interlacing" {
          tunnel: "Green laser mode" -> [_ w1451]
          tunnel: [enum32{"Laser ON", "Laser OFF", "Interlace"}."Laser OFF" ("Green laser mode") w1451] -> w1436
          tunnel: [FALSE w1447] -> w1435
          frame False {
          }
          frame True {
            n1070 = local read "Green FB On/Off"() -> (w1448:bool)
            n1071 = Equal?(x=w1451, y=enum32{"Laser ON", "Laser OFF", "Interlace"}."Interlace") -> (x = y?=w1449:bool)
            n1072 = And(x=w1449, y=w1448) -> (x .and. y?=w1447:bool)
          }
        }
        n1073 = case shown="True" "Red Laser ON/Interlacing" {
          tunnel: "Green laser mode" -> [_ w1442]
          tunnel: [FALSE w1443] -> _
          tunnel: [enum32{"Laser ON", "Laser OFF", "Interlace"}."Laser OFF" ("Green laser mode") w1442] -> w1431
          frame False {
          }
          frame True {
            n1074 = Equal?(x=w1442, y=enum32{"Laser ON", "Laser OFF", "Interlace"}."Interlace") -> (x = y?=w1443:bool)
          }
        }
        n1075 = xnode "Read/Write Control"("FPGA VI Reference In"=w1439, "error in"=w1437, "Operating Mode"=w1436, "Operating Mode 2"=w1436, "Green FB On/Off"=w1435, "Red operating mode"=w1431, "RI operating mode 2"=w1431) -> ("error out"=w1438:errorcluster)  [unwired: 1 out]
      }
      event "Green Laser ON/OFF": Value Change {
        n1076 = event-data() -> ()  [unwired: 7 out]
        n1077 = property on="Green ON/Interlacing" class="Bool (strict)"("Val(Sgnl)"="Green Laser ON/OFF") -> ()  [unwired: 2 in, 2 out]
      }
      event "Test ttrig": Value Change {
        n1078 = event-data() -> ()  [unwired: 7 out]
        n1079 = xnode "Read/Write Control"("FPGA VI Reference In"=w1456, "error in"=w1455, "TTrig?"=TRUE) -> ("error out"=w1454:errorcluster)  [unwired: 1 out]
      }
      event "Neg. TTrig FPGA": Value Change {
        n1080 = event-data() -> ()  [unwired: 7 out]
        n1081 = xnode "Read/Write Control"("FPGA VI Reference In"=w1460, "error in"=w1459, "TTrig Negate Pos"="Neg. TTrig FPGA") -> ()  [unwired: 2 out]
      }
      event "- phase (APD 1 Gate)", "+ phase (APD 1 Gate)": Value Change {
        n1082 = event-data() -> ()  [unwired: 7 out]
        n1083 = local read "Phase Adj. (APD 1 Gate)"() -> (w1461:i16)
        n1084 = Negate(x=w1461) -> (-x=w1469:i16)
        n1085 = Select(t=w1469, s="- phase (APD 1 Gate)", f=w1461) -> (s? t:f=w1468:i16)
        n1086 = Or(x="- phase (APD 1 Gate)", y="+ phase (APD 1 Gate)") -> (x .or. y?=w1464:bool)
        n1087 = xnode "Read/Write Control"("FPGA VI Reference In"=w1471, "error in"=w1470, "Phase count adjustment (APD 1 Gate)"=w1468) -> ("FPGA VI Reference Out"=w1466:T19, "error out"=w1467:errorcluster)
